vi "Update Step State.vi"(8 "error in (no error)":errorcluster, 10 "Current Time":timestamp, 11 "Output Sequencer in":refnum<class "Output Sequencer.lvclass">) -> (0 "error out":errorcluster, 3 "Output Sequencer out":refnum<class "Output Sequencer.lvclass">)   [LabVIEW 2020, in "Output Sequencer.lvlib" / "Output Sequencer.lvclass"]
uses:
  Output Sequencer.lvclass
  Output Sequencer.lvclass/Output Sequencer.ctl
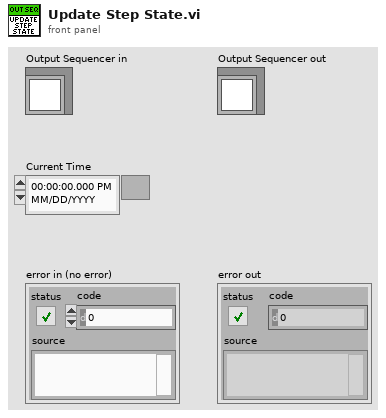
[diagram p1: front panel]
types:
  T1 = typedef "Output Sequencer.lvlib/Output Sequencer.lvclass/Sequencer State.ctl" = enum16{"Error", "Initialize", "Prepare channels", "Wait for test", "Wait for %.1f sec", "Wait for trigger", "Stop condition", "Wait for resume", "Running", "Paused", "No valid step", "Stopped"}
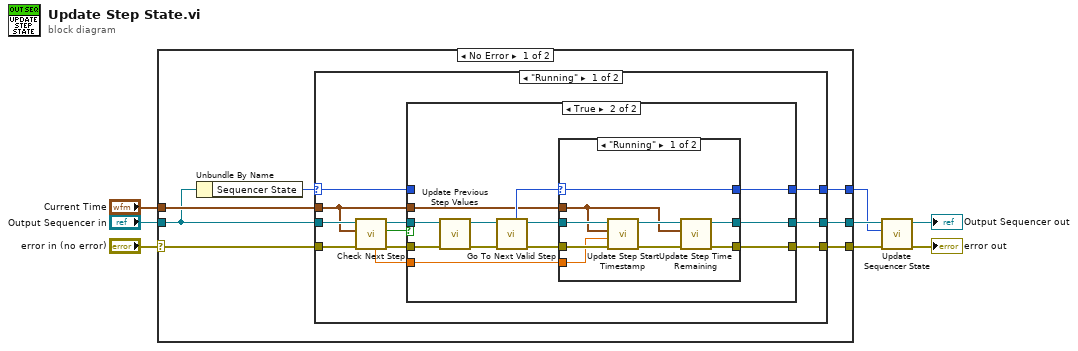
[diagram p0: block diagram]
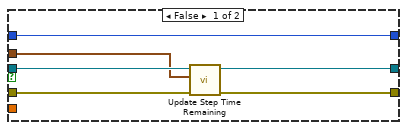
[diagram p2: hidden frame]
diagram:
  n1 = case shown="No Error" "error in (no error)" {
    selector: "error in (no error)" -> [w9 w61]
    tunnel: [w15 _] -> w1
    tunnel: "Current Time" -> [w14 _]
    tunnel: "Output Sequencer in" -> [w13 w60]
    tunnel: [w12 w61] -> w5
    tunnel: [w11 w60] -> w2
    frame No Error {
      n2 = Unbundle By Name(w13) -> ("Sequencer State"=w10:T1)
      n3 = case shown="\"Running\"" w10 {
        selector: w10 -> [w17 w57]
        tunnel: [w26 w59] -> w11
        tunnel: w14 -> [w19 _]
        tunnel: w13 -> [w24 w59]
        tunnel: w9 -> [w23 w58]
        tunnel: [w25 w58] -> w12
        tunnel: [w16 w57] -> w15
        frame "Running" {
          n4 = call "Check Next Step.vi"("error in (no error)"=w23, "Current Time"=w19, "Output Sequencer in"=w24) -> ("error out"=w21:errorcluster, "Go to Next Step"=w20:bool, "Output Sequencer out"=w22:refnum<class "Output Sequencer.lvclass">, "Current Step End Timestamp"=w18:dbl)  [unwired: 5 in]
          n5 = case shown="True" w20 {
            tunnel: w22 -> [w30 w42]
            tunnel: [w32 w44] -> w26
            tunnel: w18 -> [_ w43]
            tunnel: w21 -> [w29 w41]
            tunnel: [w31 w40] -> w25
            tunnel: w19 -> [w28 w33]
            tunnel: w17 -> [w27 _]
            tunnel: [w27 w34] -> w16
            frame False {
              n6 = call "Update Step Time Remaining.vi"("error in (no error)"=w29, "Current Time"=w28, "Output Sequencer in"=w30) -> ("error out"=w31:errorcluster, "Output Sequencer out"=w32:refnum<class "Output Sequencer.lvclass">)  [unwired: 7 in]
            }
            frame True {
              n7 = call "Update Previous Step Values.vi"("error in (no error)"=w41, "Output Sequencer in"=w42) -> ("error out"=w38:errorcluster, "Output Sequencer out"=w39:refnum<class "Output Sequencer.lvclass">)  [unwired: 8 in]
              n8 = call "Go To Next Valid Step.vi"("error in (no error)"=w38, "Output Sequencer in"=w39) -> ("error out"=w37:errorcluster, "Output Sequencer out"=w36:refnum<class "Output Sequencer.lvclass">, "Sequencer State"=w35:T1)  [unwired: 7 in]
              n9 = case shown="\"Running\"" w35 {
                selector: w35 -> [w45 w54]
                tunnel: w36 -> [w51 w55]
                tunnel: w37 -> [w50 w56]
                tunnel: w33 -> [w49 _]
                tunnel: w43 -> [w48 _]
                tunnel: [w47 w55] -> w44
                tunnel: [w46 w56] -> w40
                tunnel: [w45 w54] -> w34
                frame "Running" {
                  n10 = call "Update Step Start Timestamp.vi"("error in (no error)"=w50, "Previous step end timestamp"=w48, "Current Time"=w49, "Output Sequencer in"=w51) -> ("error out"=w53:errorcluster, "Output Sequencer out"=w52:refnum<class "Output Sequencer.lvclass">)  [unwired: 6 in]
                  n11 = call "Update Step Time Remaining.vi"("error in (no error)"=w53, "Current Time"=w49, "Output Sequencer in"=w52) -> ("error out"=w46:errorcluster, "Output Sequencer out"=w47:refnum<class "Output Sequencer.lvclass">)  [unwired: 7 in]
                }
                frame Default {
                }
              }
            }
          }
        }
        frame Default {
        }
      }
    }
    frame Error {
    }
  }
  n12 = call "Update Sequencer State.vi"("error in (no error)"=w5, "Sequencer State"=w1, "Output Sequencer in"=w2) -> ("error out"=→"error out":errorcluster, "Output Sequencer out"=→"Output Sequencer out":refnum<class "Output Sequencer.lvclass">)  [unwired: 7 in]
